vi "paramToTS.vi"(11 "dataout":u32[](array[numeric]) format="%x") -> (1 "numberSignals":u32, 2 "resolution":u32, 3 "readyData":u32[](array[numeric])=[10, 10, 10, 10, 10, 10, 10, 10, 10, 10, 10, 10, 10, 10, 10, 10, 4294967295, 0, 4294967295, 0, 4294967295, 0, 4294967295, 0, 4294967295, 0, 4294967295, 0, 4294967295, 0, 4294967295, 0, 65535] format="%x")   [LabVIEW 2014]
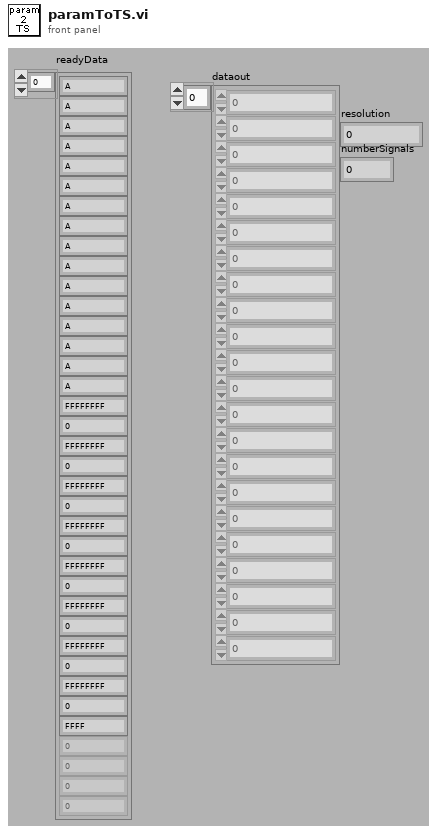
[diagram p1: front panel]
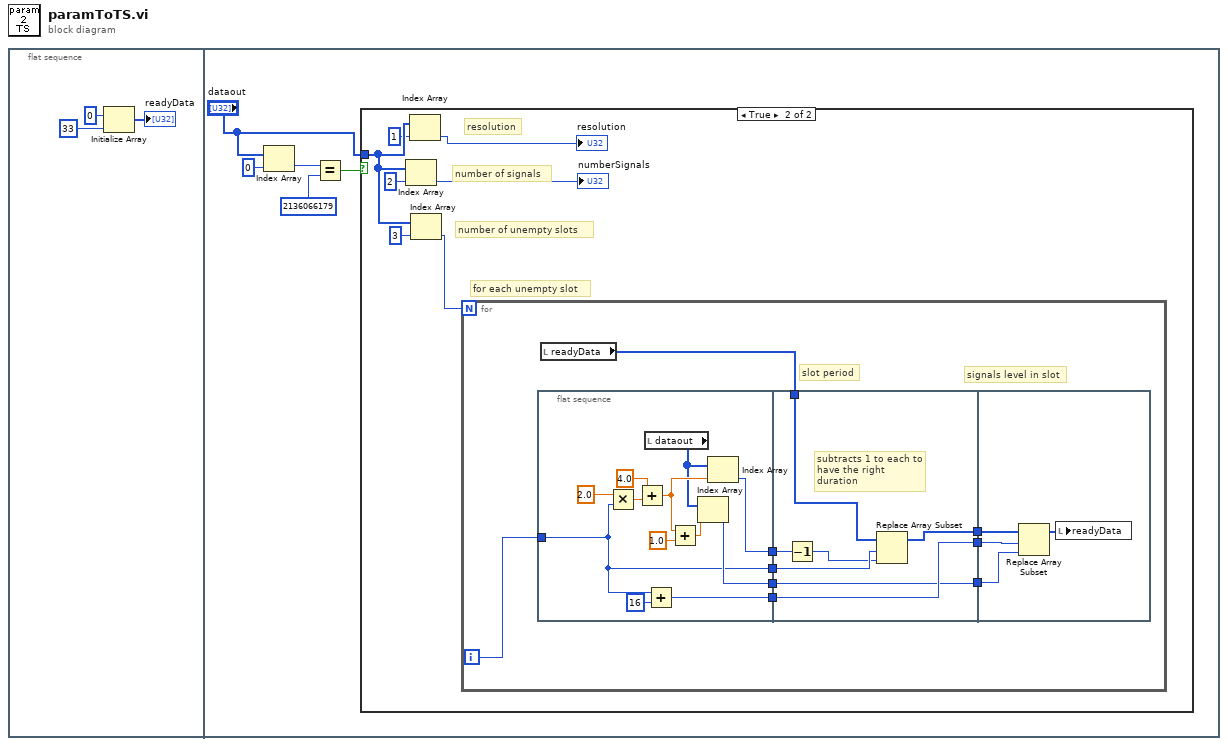
[diagram p0: block diagram]
diagram:
  n1 = flat-sequence {
    frame #0 {
      n2 = Initialize Array(u32 0 ("element"), 33 ("dimension size")) -> (→"readyData":u32[])
    }
    frame #1 {
      n3 = Index Array(array="dataout", index=0) -> (element=w6:u32)
      n4 = Equal?(x=w6, y=u32 2136066179) -> (x = y?=w7:bool)
      n5 = case shown="True" w7 {
        tunnel: "dataout" -> [_ w12]
        frame False {
        }
        frame True {
          # "resolution"
          # "for each unempty slot"
          # "number of unempty slots"
          # "number of signals"
          n6 = Index Array(array=w12, index=2) -> (element=→"numberSignals":u32)
          n7 = Index Array(array=w12, index=1) -> (element=→"resolution":u32)
          n8 = Index Array(array=w12, index=3) -> (element=w13:u32)
          n9 = for {
            N: w13 -> [_]
            i -> [w23]
            # "signals level in slot"
            # "slot period"
            n10 = flat-sequence {
              tunnel: w23 -> [w25]
              tunnel: [w28] -> w22
              tunnel: [w27] -> w20
              tunnel: [w26] -> w18
              tunnel: [w25] -> w17
              tunnel: [w43] -> w24
              tunnel: w22 -> [w42]
              tunnel: [w42] -> w21
              tunnel: w20 -> [w41]
              tunnel: [w40] -> w19
              tunnel: w18 -> [w40]
              tunnel: w17 -> [w39]
              tunnel: w16 -> [w38]
              tunnel: w24 -> [w46]
              tunnel: w21 -> [w45]
              tunnel: w19 -> [w44]
              frame #0 {
                n11 = Multiply(x=2.0 ("y"), y=w25) -> (x*y=w32:dbl)
                n12 = Add(x=w32, y=4.0) -> (x+y=w34:dbl)
                n13 = local read "dataout"() -> (w29:u32[])
                n14 = Add(x=w25, y=16) -> (x+y=w28:i32)
                n15 = Add(x=w34, y=1.0) -> (x+y=w31:dbl)
                n16 = Index Array(array=w29, index=w31) -> (element=w26:u32)
                n17 = Index Array(array=w29, index=w34) -> (element=w27:u32)
              }
              frame #1 {
                # "subtracts 1 to each to have the right duration"
                n18 = Decrement(x=w41) -> (x-1=w37:u32)
                n19 = Replace Array Subset(array=w38, new element=w37, index=w39) -> (w43:u32[])
              }
              frame #2 {
                n20 = Replace Array Subset(array=w46, new element=w44, index=w45) -> (w47:u32[])
                n21 = local write "readyData"(w47) -> ()
              }
            }
            n22 = local read "readyData"() -> (w16:u32[])
          }
        }
      }
    }
  }
